vi "USB_Relay_On_Off_Relay.vi"(2 "error in (no error)":errorcluster, 3 "Channel":u16 format="%02.0f", 4 "ON/OFF":bool, 5 "Module Name":string="BITFT") -> (0 "error out":errorcluster, 1 "OK":bool)   [LabVIEW 2016]
panel:
  out "Cmd":string
  out "standard error":string
  out "standard output":string
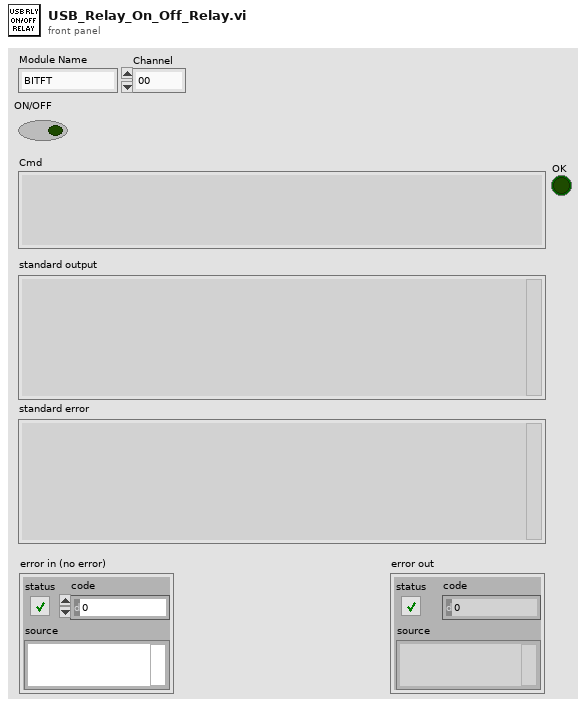
[diagram p1: front panel]
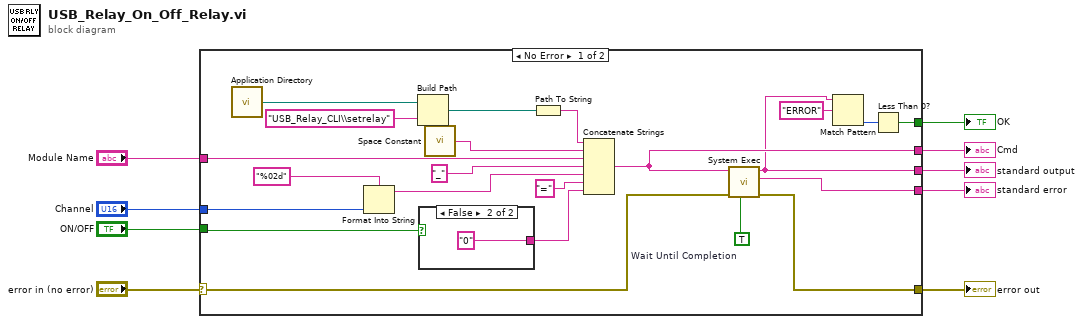
[diagram p0: block diagram]
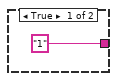
[diagram p2: hidden frame]
diagram:
  n1 = case shown="No Error" "error in (no error)" {
    selector: "error in (no error)" -> [w28 w34]
    tunnel: [w11 _] -> w9
    tunnel: [w31 _] -> w8
    tunnel: [w30 w34] -> w7
    tunnel: [w27 _] -> w5
    tunnel: "ON/OFF" -> [w24 _]
    tunnel: "Channel" -> [w19 _]
    tunnel: "Module Name" -> [w21 _]
    tunnel: [w10 _] -> w1
    frame No Error {
      w29 = TRUE  # Wait Until Completion
      n2 = call <vilib>:"Application Directory.vi"() -> ("Application Directory"=w18:path)
      n3 = Format Into String(format string="%02d", w19) -> (resulting string=w15:string)  [unwired: 2 in, 1 out]
      n4 = Build Path(base path=w18, name or relative path="USB_Relay_CLI\\setrelay") -> (appended path=w26:path)
      n5 = case shown="False" w24 {
        tunnel: ["1" "0"] -> w16
        frame True {
        }
        frame False {
        }
      }
      n6 = call <vilib>:"Space Constant.vi"() -> ("String"=w22:string)
      n7 = Path To String(path=w26) -> (string=w23:string)
      n8 = Concatenate Strings(w23, w22, w21, "_" ("string"), w15, "=" ("string"), w16) -> (w27:string)
      n9 = call <vilib>:"System Exec.vi"("run minimized? (F)"=w29, "error in (no error)"=w28, "command line"=w27) -> ("error out"=w30:errorcluster, "standard error"=w31:string, "standard output"=w11:string)  [unwired: 5 in, 1 out]
      n10 = Match Pattern(string=w11, regular expression="ERROR") -> (offset past match=w13:i32)  [unwired: 1 in, 3 out]
      n11 = Less Than 0?(x=w13) -> (x < 0?=w10:bool)
    }
    frame Error {
    }
  }
  "standard output" <- w9
  "standard error" <- w8
  "error out" <- w7
  "Cmd" <- w5
  "OK" <- w1
